vi "Evaluate Scope.vi"(11 "cluster":T1) -> (3 "dataflow out":T1)   [LabVIEW 2024, in "Logging.lvlib" / "Logger.lvclass"]
uses:
  Logger.lvclass
  Logger.lvclass/Logger.ctl
  056461df-8a4d-4d26-9c91-3850ac14247b.vi
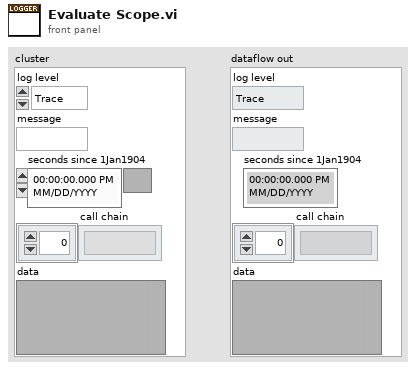
[diagram p1: front panel]
types:
  T1 = cluster{"log level":enum16{"Trace", "Debug", "Info", "Warning", "Error", "Critical"}, "message":string, "seconds since 1Jan1904":timestamp, "call chain":string[], "data":variant}
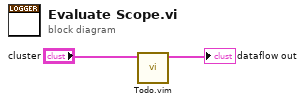
[diagram p0: block diagram]
diagram:
  n1 = call "Todo.vim"("dataflow in"="cluster") -> ("dataflow out"=→"dataflow out":T1)  [unwired: 10 in]
